vi "User Logic.vi"(7 "read data shift reg":u64, 9 "read data valid":bool, 11 "read bit status":T1) -> (10 "useful reg":u64, 15 "data to master":u64)   [LabVIEW 2013, in "DIO SPI User Library.lvlib"]
doc: "This slave code interfaces with the SPI Slave to provide an example of how standard SPI slave logic might be implemented in LabVIEW FPGA. This code contains a set of readable and writable registers that can be accessed through SPI. The first eight bits of a SPI transaction determine whether the transaction is a read or a write and what register offset is being accessed."
uses:
  DIO SPI User Library.lvlib
  Perforce/MI/Apps/IP/SPI/trunk/1.1/source/LV/user.lib/._NI SPI IP/FPGA/Controllers/Public/Read Bit Status.ctl
panel:
  # "This slave code interfaces with the SPI Slave to provide an example of how standard SPI slave logic might be implemented in LabVIEW FPGA. This code contains a set of readable and writable registers that can be accessed through SPI. The first eight bits of a SPI transaction determine whether the transaction is a read or a write and what register offset is being accessed."
  # "From SPI Slave"
  # "Example Output"
  # "To SPI Slave"
  # "This output is simply an example that data can be ready outside of this VI."
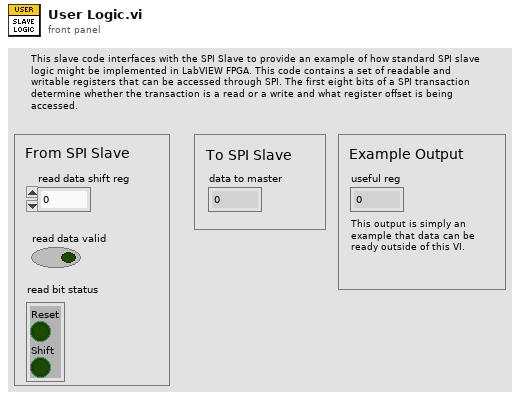
[diagram p1: front panel]
types:
  T1 = typedef "DIO SPI FPGA.lvlib/Read Bit Status.ctl" = cluster{"Reset":bool, "Shift":bool}
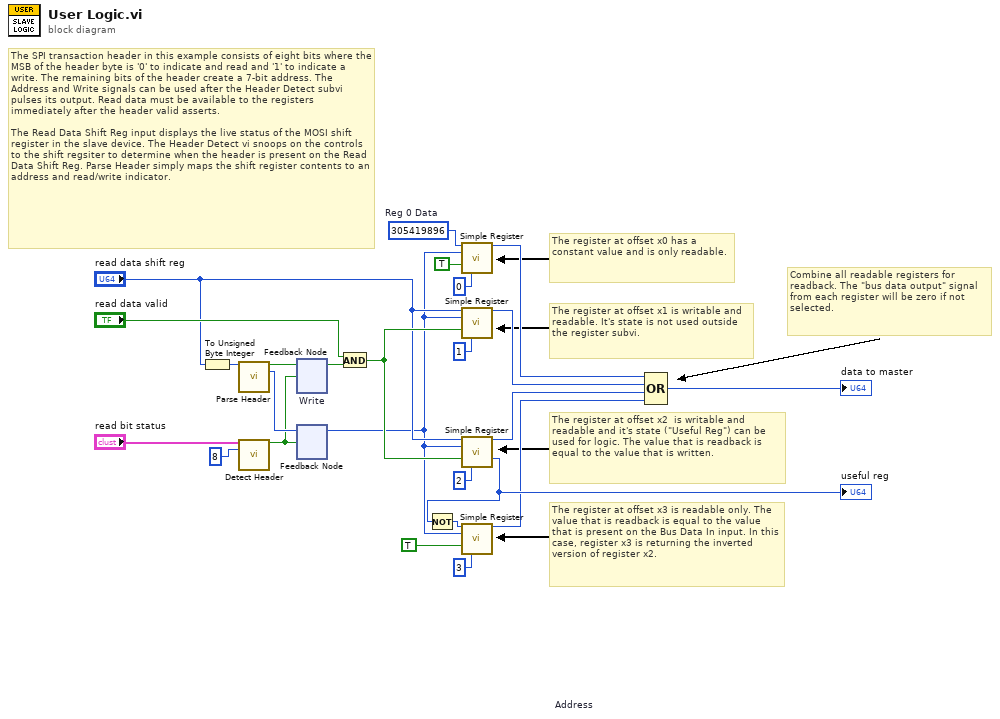
[diagram p0: block diagram]
diagram:
  w18 = u64 305419896  # Reg 0 Data
  # "Combine all readable registers for readback. The \"bus data output\" signal from each register will be zero if not selected."
  # "The register at offset x3 is readable only. The value that is readback is equal to the value that is present on the Bus Data In input. In this case, register x3 is returning the inverted version of register x2."
  # "The register at offset x2  is writable and readable and it's state (\"Useful Reg\") can be used for logic. The value that is readback is equal to the value that is written."
  # "The register at offset x1 is writable and readable. It's state is not used outside the register subvi."
  # "The register at offset x0 has a constant value and is only readable."
  # "The SPI transaction header in this example consists of eight bits where the MSB of the header byte is '0' to indicate and read and '1' to indicate a write. The remaining bits of the header create a 7-bit address. The Address and Write signals can be used after the Header Detect subvi pulses its output. Read data must be available to the registers immediately after the header valid asserts.\n\nThe Read Data Shift Reg input displays the live status of the MOSI shift register in the slave device. The Header Detect vi snoops on the controls to the shift regsiter to determine when the header is present on the Read Data Shift Reg. Parse Header simply maps the shift register contents to an address and read/write indicator."
  n1 = To Unsigned Byte Integer(number="read data shift reg") -> (unsigned 8bit integer=w25:u8)
  n2 = call "Parse Header.vi"("header in"=w25) -> ("write"=w24:bool, "address"=w23:u8)  [unwired: 13 in]
  n3 = call "Detect Header.vi"("read bit status"="read bit status", "header size"=u8 8 ("HeaderSize")) -> ("header valid"=w11:bool)  [unwired: 13 in]
  n4 = feedback #1 "Write"() -> (w22:bool)  [unwired: 1 in]
  n5 = feedback-in #1(w24, w11) -> ()
  n6 = feedback #2 "Address"() -> (w4:u8)  [unwired: 1 in]
  n7 = feedback-in #2(w23, w11) -> ()
  n8 = And(x="read data valid", y=w22) -> (x .and. y?=w9:bool)
  n9 = call "Simple Register.vi"("bus data input"=w18, "bus address"=w4, "bus write pulse"=TRUE ("Bus Write Pulse"), "register offset"=u8 0 ("Register Offset")) -> ("bus data output"=w16:u64)  [unwired: 10 in, 1 out]
  n10 = call "Simple Register.vi"("bus data input"="read data shift reg", "bus address"=w4, "bus write pulse"=w9, "register offset"=u8 1 ("Register Offset")) -> ("bus data output"=w15:u64)  [unwired: 10 in, 1 out]
  n11 = call "Simple Register.vi"("bus data input"="read data shift reg", "bus address"=w4, "bus write pulse"=w9, "register offset"=u8 2 ("Register Offset")) -> ("bus data output"=w8:u64, "register contents"=w3:u64)  [unwired: 10 in]
  "useful reg" <- w3
  n12 = Not(x=w3) -> (.not. x?=w2:u64)
  n13 = call "Simple Register.vi"("bus data input"=w2, "bus address"=w4, "bus write pulse"=TRUE ("Bus Write Pulse"), "register offset"=u8 3 ("Register Offset")) -> ("bus data output"=w1:u64)  [unwired: 10 in, 1 out]
  n14 = Compound Arithmetic op=OR(w16, w15, w8, w1) -> (→"data to master":u64)
